vi "Read.vi"(0 "MB class in":refnum<class "MB class.lvclass">, 5 "Address":T1, 7 "startReg":u16, 9 "Quantity":u16=1, 11 "error in (no error)":errorcluster) -> (4 "MB class out":refnum<class "MB class.lvclass">, 8 "Holding Registers":u16[](array[numeric]), 10 "Numeric":i16, 15 "error out":errorcluster)   [LabVIEW 2020, in "MB class.lvclass"]
uses:
  MB class.lvclass
  MB class.lvclass/MB class.ctl
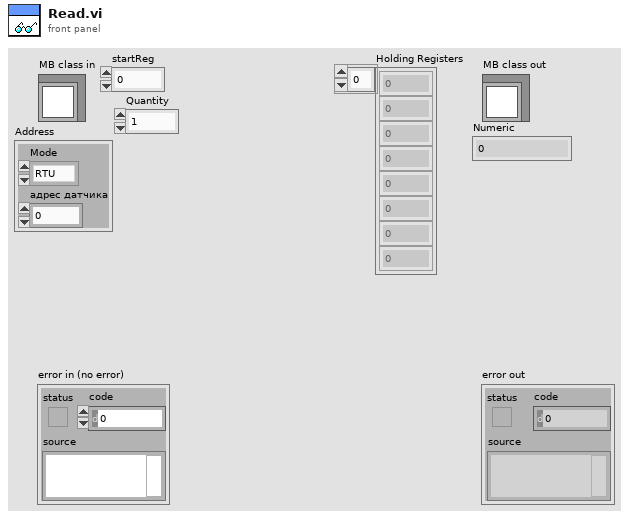
[diagram p1: front panel]
types:
  T1 = cluster{"Mode":enum16{"RTU", "ASCII"}, "адрес датчика":u16}
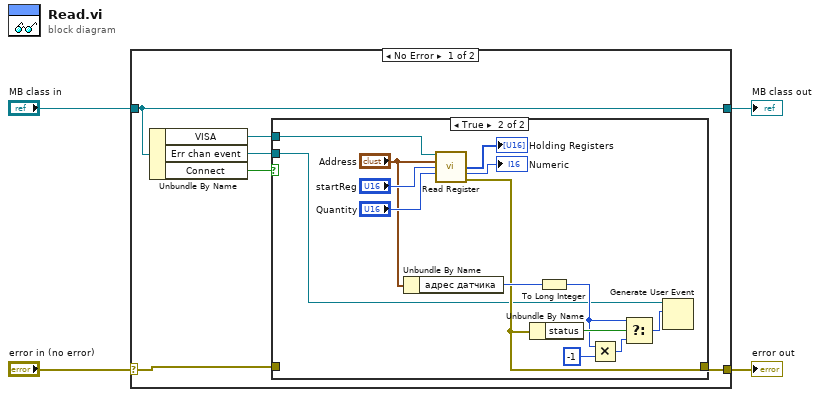
[diagram p0: block diagram]
diagram:
  n1 = case shown="No Error" "error in (no error)" {
    selector: "error in (no error)" -> [w5 w27]
    tunnel: [w8 w27] -> w3
    tunnel: [w10 w26] -> w1
    tunnel: "MB class in" -> [w10 w26]
    frame No Error {
      n2 = Unbundle By Name(w10) -> ("VISA"=w9:refnum<visa-resource-name>, "Err chan event"=w7:refnum<user-event>, "Connect"=w6:bool)
      n3 = case shown="True" w6 {
        tunnel: w9 -> [_ w25]
        tunnel: [w11 w13] -> w8
        tunnel: w7 -> [_ w12]
        tunnel: w5 -> [w11 _]
        frame False {
        }
        frame True {
          n4 = Unbundle By Name("Address") -> ("адрес датчика"=w14:u16)
          n5 = call "Read Register.vi"("Refnum in"=w25, "Mode"="Address", "startReg"="startReg", "Quantity"="Quantity") -> ("Holding Registers"=→"Holding Registers":u16[], "Numeric"=→"Numeric":i16, "error out"=w13:errorcluster)  [unwired: 7 in, 2 out]
          n6 = Unbundle By Name(w13) -> ("status"=w19:bool)
          n7 = To Long Integer(number=w14) -> (32bit integer=w17:i32)
          n8 = Multiply(x=w17, y=-1) -> (x*y=w15:i32)
          n9 = Select(t=w17, s=w19, f=w15) -> (s? t:f=w18:i32)
          n10 = Generate User Event(user event=w12, event data cluster=w18) -> ()  [unwired: 2 in, 2 out]
        }
      }
    }
    frame Error {
    }
  }
  "error out" <- w3
  "MB class out" <- w1
